vi "Arm Motor.vi"(6 "Stall Arm?":bool, 8 "Mode":enum16{"Init", "Run", "End"}(ring), 9 "Arm motor speed":dbl, 11 "PWM Module (DIO A)":T1={"PWM Module"=enum."Digital Module 2", "Unassigned"=enum."PWM 1", "Unassigned"=enum."PWM 2", "Right Motor"=enum."PWM 3", "Left Motor"=enum."PWM 4", "Unassigned"=enum."PWM 5", "Unassigned"=enum."PWM 6", "Unassigned"=enum."PWM 7", "Arm Motor"=enum."PWM 8", "Unassigned"=enum."PWM 9", "Unassigned"=enum."PWM 10", "Compressor"=enum."Relay 1", "Unassigned"=enum."Relay 2", "Unassigned"=enum."Relay 3", "Unassigned"=enum."Relay 4", "Unassigned"=enum."Relay 5", "Unassigned"=enum."Relay 6", "Unassigned"=enum."Relay 7", "Unassigned "=enum."Relay 8"}) -> ()   [LabVIEW 2013]
doc: "Set the Arm Motor"
uses:
  Type Defs/PWM Module (DIO A).ctl
  <vilib>/Rock Robotics/SystemInterfaces/Typedef/FPGA_TypedefDigitalModule.ctl
  <vilib>/Rock Robotics/SystemInterfaces/DIO/FPGA_DIOPWMChannel.ctl
  <vilib>/Rock Robotics/SystemInterfaces/DIO/FPGA_DIORelayChannel.ctl
  <vilib>/Rock Robotics/WPI/SafetyOutput/WPI_SafetyOutputConfigMenu.ctl
  <vilib>/Rock Robotics/WPI/MotorControl/WPI_MotorControlOpen Victor.vi
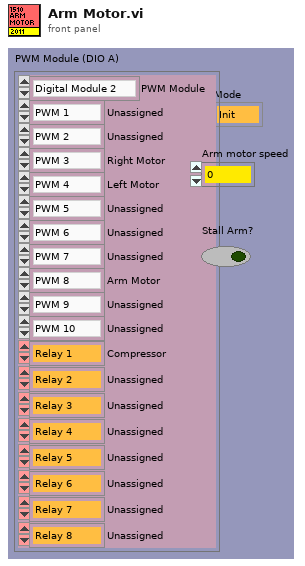
[diagram p1: front panel]
types:
  T1 = typedef "PWM Module (DIO A).ctl" = cluster{"PWM Module":T2, "Unassigned":T3, "Unassigned":T3, "Right Motor":T3, "Left Motor":T3, "Unassigned":T3, "Unassigned":T3, "Unassigned":T3, "Arm Motor":T3, "Unassigned":T3, "Unassigned":T3, "Compressor":T4, "Unassigned":T4, "Unassigned":T4, "Unassigned":T4, "Unassigned":T4, "Unassigned":T4, "Unassigned":T4, "Unassigned ":T4}
  T2 = typedef "FPGA_TypedefDigitalModule.ctl" = enum16{"Digital Module 1", "Digital Module 2"}
  T3 = typedef "FPGA_DIOPWMChannel.ctl" = enum8{"PWM 1", "PWM 2", "PWM 3", "PWM 4", "PWM 5", "PWM 6", "PWM 7", "PWM 8", "PWM 9", "PWM 10", "Invalid"}
  T4 = typedef "FPGA_DIORelayChannel.ctl" = enum8{"Relay 1", "Relay 2", "Relay 3", "Relay 4", "Relay 5", "Relay 6", "Relay 7", "Relay 8", "Invalid"}
  T5 = typedef "WPI_SafetyOutputConfigMenu.ctl" = enum16{"Enable", "Disable"}
  T6 = typedef "WPI_MotorControlDeviceRef.ctl" = cluster{"DeviceStatus":errorcluster, "Type":enum16{"PWM", "CAN"}, "PWM":cluster{"Digital Module":T2, "PWM Channel":T3, "DeadBand":T7}, "CAN":cluster{"Device Number":u8, "Control Mode":T8, "Semaphore":T9, "Max Vout":dbl}, "Invert":bool, "TransformRef":T10, "InvTransformRef":T10}
  T7 = typedef "WPI_PWMDeadband.ctl" = cluster{"Name":string, "maxPositivePwm":i32, "minPositivePwm":i32, "centerPwm":i32, "maxNegativePwm":i32, "minNegativePwm":i32, "angularRange":u16}
  T8 = typedef "WPI_CANJaguar_ControlMode.ctl" = enum8{"Percent VBus", "Current", "Speed", "Position", "Voltage"}
  T9 = typedef "Semaphore RefNum" = refnum<k1>
  T10 = typedef "WPI_PWMTransform_ConPane.ctl" = refnum<vi>
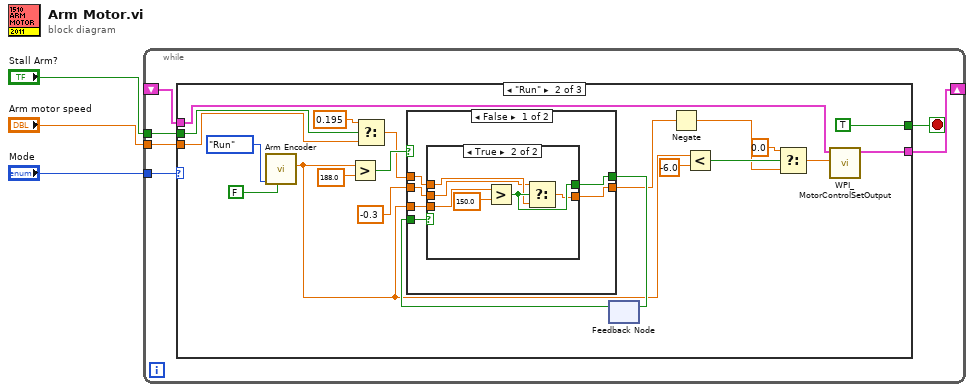
[diagram p0: block diagram]
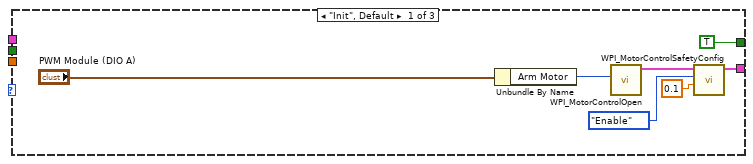
[diagram p2: hidden frame]
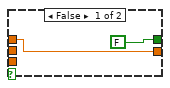
[diagram p3: hidden frame]
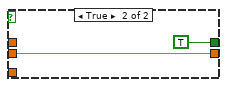
[diagram p4: hidden frame]
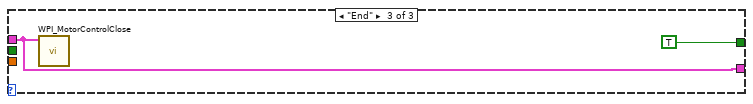
[diagram p5: hidden frame]
diagram:
  n1 = while {
    tunnel: "Mode" -> [w9]
    shift-right: [w8] -> _
    shift-left: _ -> [w7]
    tunnel: "Arm motor speed" -> [w5]
    tunnel: "Stall Arm?" -> [w4]
    stop <- w6 stop-if-true
    n2 = case shown="\"Run\"" w9 {
      tunnel: [w12 w36 w54] -> w8
      tunnel: w7 -> [_ w35 w54]
      tunnel: [TRUE TRUE TRUE] -> w6
      tunnel: w5 -> [_ w18 _]
      tunnel: w4 -> [_ w22 _]
      frame "Init", Default {
        n3 = Unbundle By Name("PWM Module (DIO A)") -> ("Arm Motor"=w14:T3)
        n4 = call-poly <vilib>:"WPI_MotorControlOpen.vi"("PWM Channel"=w14) -> ("MotorControlDeviceRef"=w13:T6)  [unwired: 6 in, 4 out]
        n5 = call <vilib>:"WPI_MotorControlSafetyConfig.vi"("timeout (s)"=0.1, "mode"=WPI_SafetyOutputConfigMenu."Enable", "MotorControlDevRef"=w13) -> ("MotorControlDevRef"=w12:T6)  [unwired: 1 in, 7 out]
      }
      frame "Run" {
        n6 = call "Arm Encoder.vi"("Reset Encoder?"=FALSE, "Mode"=enum16{"Init", "Run", "End"}."Run") -> ("Get Arm Encoder"=w27:dbl)  [unwired: 1 in, 8 out]
        n7 = Greater?(x=w27, y=188.0) -> (0:w29:bool)
        n8 = Select(t=0.195 ("f"), s=w22, f=w18) -> (s? t:f=w21:dbl)
        n9 = feedback #1() -> (w31:bool)  [unwired: 1 out]
        n10 = case shown="False" w29 {
          tunnel: w31 -> [w43 _]
          tunnel: [w41 TRUE] -> w32
          tunnel: w27 -> [w42 _]
          tunnel: [w40 w52] -> w28
          tunnel: w21 -> [w39 _]
          tunnel: -0.3 ("f") -> [w38 w52]
          frame False {
            n11 = case shown="True" w43 {
              tunnel: w42 -> [_ w51]
              tunnel: [FALSE w49] -> w41
              tunnel: [w45 w47] -> w40
              tunnel: w39 -> [w45 w48]
              tunnel: w38 -> [_ w46]
              frame False {
              }
              frame True {
                n12 = Greater?(x=w51, y=150.0) -> (0:w49:bool)
                n13 = Select(t=w46, s=w49, f=w48) -> (s? t:f=w47:dbl)
              }
            }
          }
          frame True {
          }
        }
        n14 = feedback-in #1(w32) -> ()
        n15 = Negate(x=w28) -> (-x=w23:dbl)
        n16 = Less?(x=w27, y=-6.0) -> (x < y?=w25:bool)
        n17 = Select(t=0.0, s=w25, f=w23) -> (s? t:f=w20:dbl)
        n18 = call <vilib>:"WPI_MotorControlSetOutput.vi"("Output"=w20, "MotorControlDevRef"=w35) -> ("MotorControlDevRef"=w36:T6)  [unwired: 3 in, 6 out]
      }
      frame "End" {
        n19 = call <vilib>:"WPI_MotorControlClose.vi"("MotorControlDevRef"=w54) -> ()  [unwired: 1 in, 10 out]
      }
    }
  }
